vi "电机定位1.1（40M只处理采集卡）.vi"(0 "VISA I":refnum<visa-resource-name>, 1 "等待时间(ms)":u32=40, 2 "细分设置":dbl=8.0, 3 "电机急停":bool, 4 "X":dbl, 5 "精度":dbl=0.001, 6 "pulDDR2Length":u32, 8 "hDevice":i32, 10 "M-length":dbl, 12 "N-length":dbl) -> (13 "hDevice out":i32, 14 "VISA O":refnum<visa-resource-name>, 18 "X":dbl, 19 "Y":dbl)   [LabVIEW 2016]
uses:
  <vilib>/Analysis/2dsp.llb/Real FFT.vi
  <vilib>/Utility/file.llb/Write Delimited Spreadsheet (DBL).vi
  <vilib>/Utility/file.llb/Read Delimited Spreadsheet (DBL).vi
  <vilib>/Analysis/NI_AALBase.lvlib
  <vilib>/Analysis/NI_AALPro.lvlib
panel:
  out "定点积分读数":dbl
  out "有效值":dbl
  out "空扫底噪":cdb[](array[numeric])
  out "采集卡底噪":cdb[](array[numeric])
  in  "保存信号":bool
  out "幅频谱":dbl[](graph)
  out "时域谱":dbl[](graph)
  in  "查询信号":bool
  in  "Y":dbl
  in  "确定":bool
  in  "ESC":bool
  # "时域谱"
  # "频域谱"
  # "目标位置"
  # "实时位置"
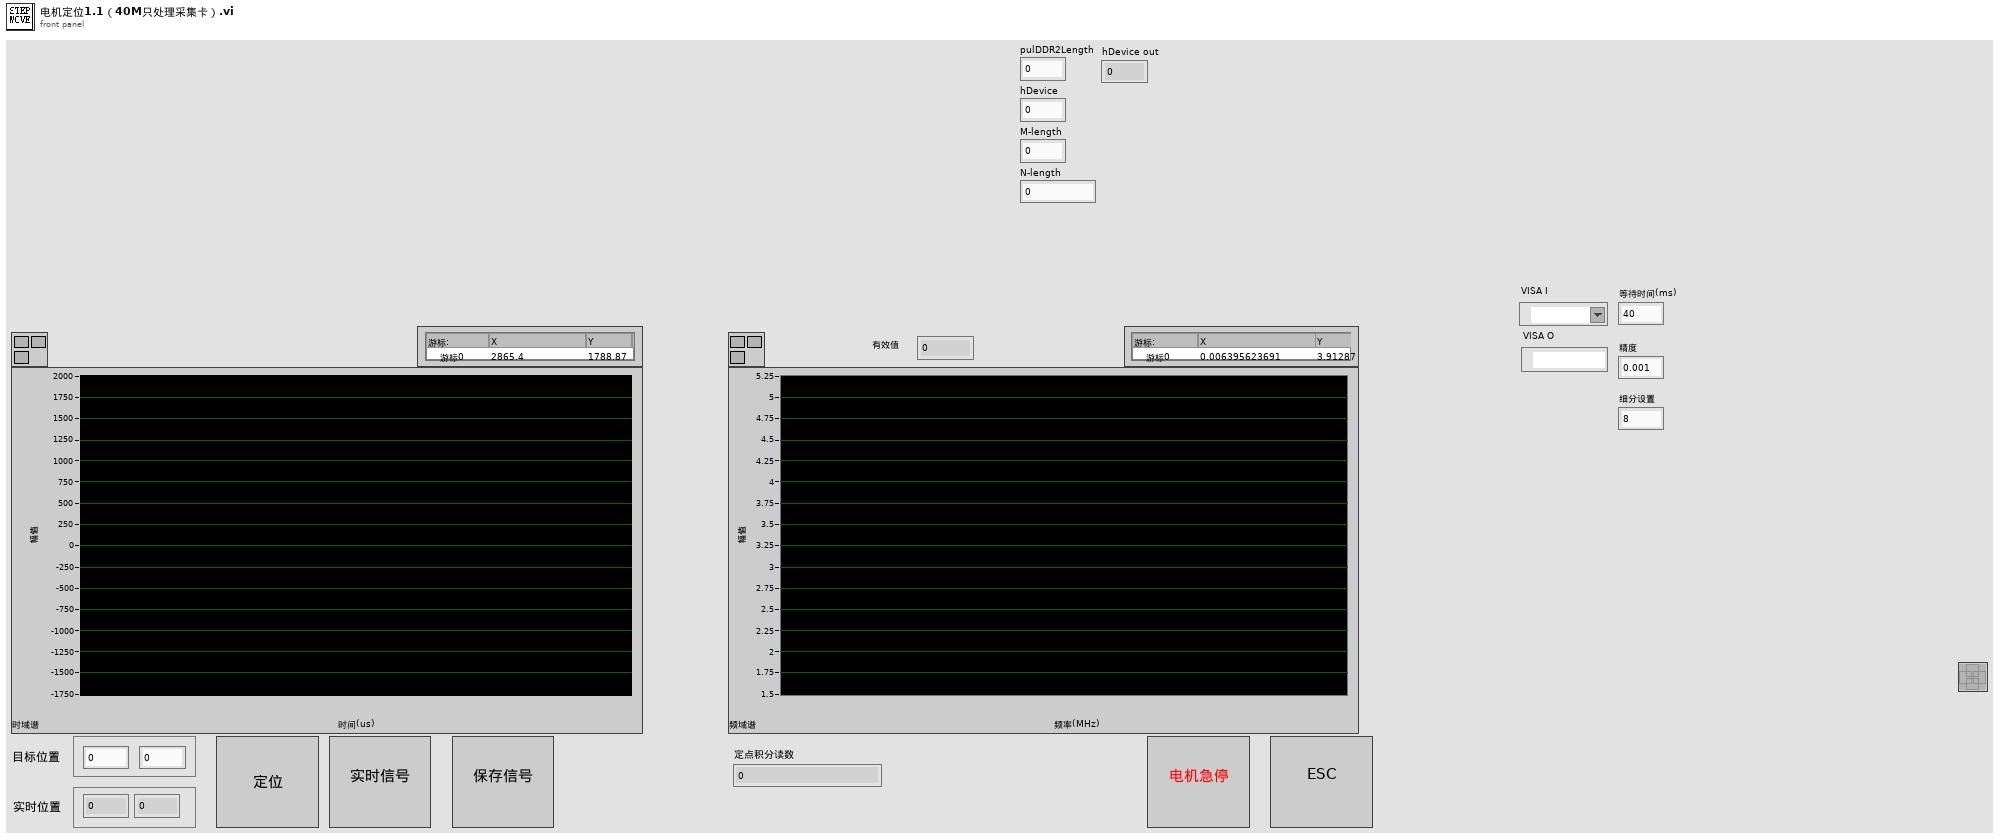
[diagram p1: front panel]
types:
  T1 = enum16{"open", "replace", "create", "open or create", "replace or create", "replace or create with confirmation"}
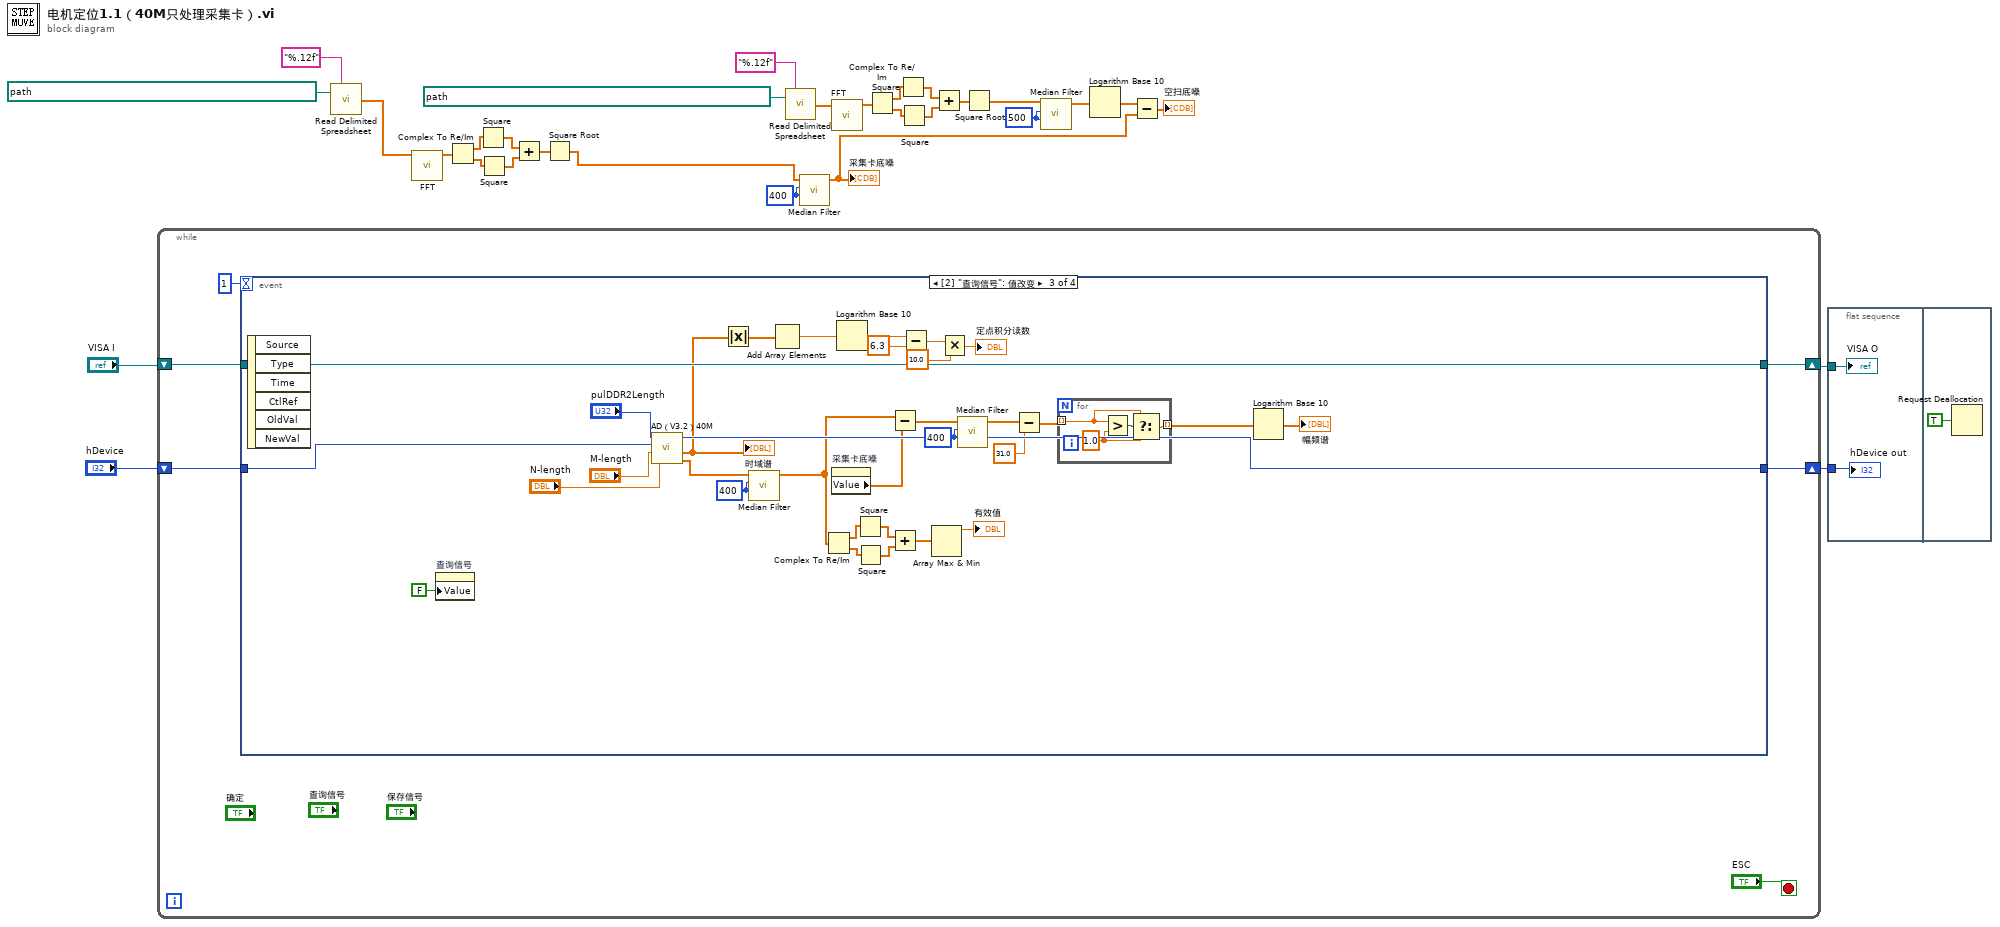
[diagram p0: block diagram]
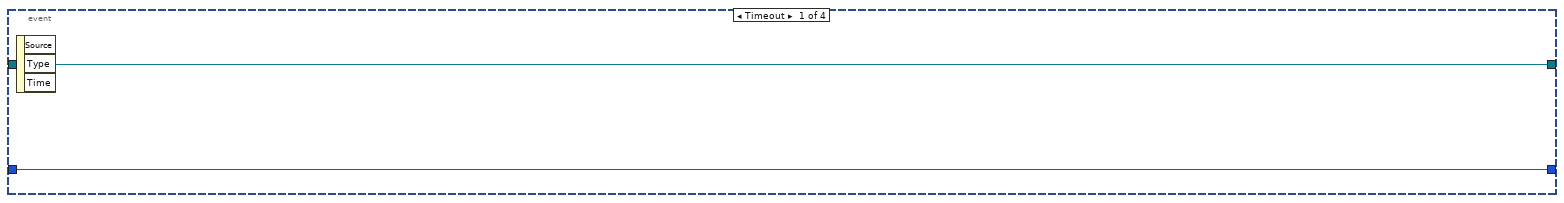
[diagram p2: hidden frame]
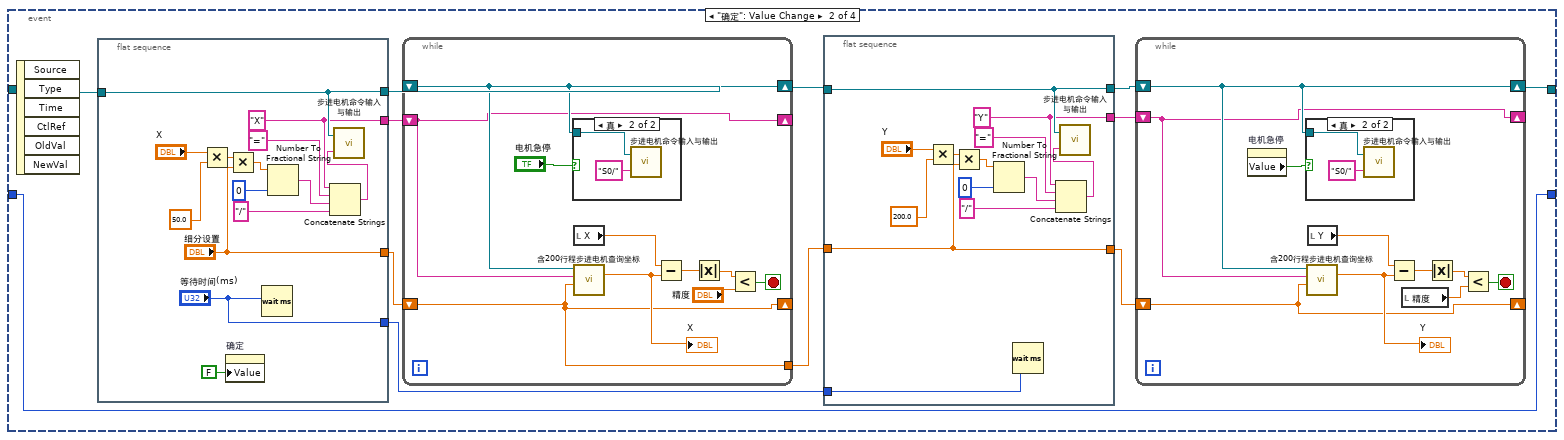
[diagram p3: hidden frame]
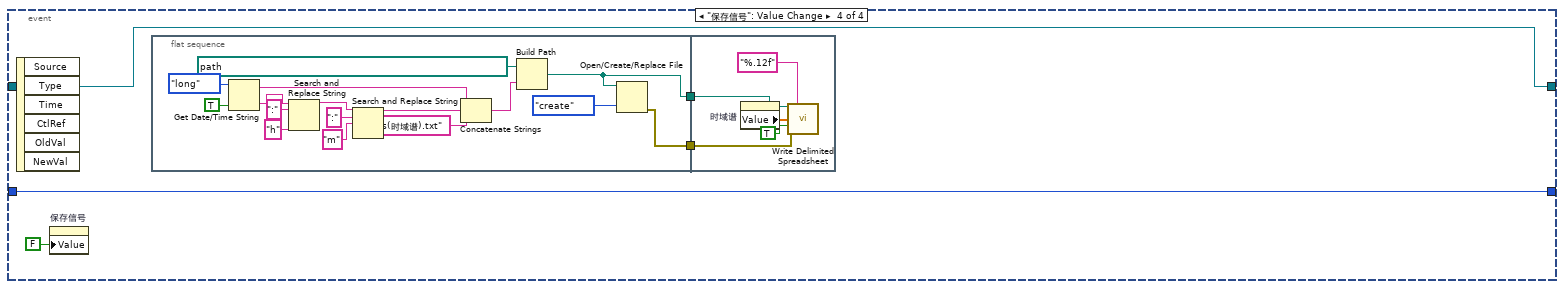
[diagram p6: hidden frame]
diagram:
  w6 = 400 ("left rank")
  w24 = 500 ("left rank")
  n1 = while {
    shift-right: [w35] -> w30
    shift-left: "VISA I" -> [w36]
    shift-right: [w32] -> w27
    shift-left: "hDevice" -> [w33]
    stop <- "ESC" stop-if-true
    n2 = event shown="[2] \"查询信号\": 值改变" {
      selector: _ -> [_ _ _ _]
      dyn-events: _ -> [_ _ _ _]
      timeout: 1 -> [_ _ _ _]
      tunnel: w36 -> [w38 w50 w133 w141]
      tunnel: [w38 w49 w133 w141] -> w35
      tunnel: w33 -> [w37 w39 w129 w140]
      tunnel: [w37 w39 w128 w140] -> w32
      event Timeout {
        n3 = event-data() -> ()  [unwired: 1 in, 3 out]
      }
      event "确定": Value Change {
        n4 = event-data() -> ()  [unwired: 1 in, 6 out]
        n5 = flat-sequence {
          tunnel: w50 -> [w93]
          tunnel: [w93] -> w48
          tunnel: ["细分设置"] -> w47
          tunnel: [w90] -> w46
          tunnel: ["等待时间(ms)"] -> w41
          frame #0 {
            w90 = "X"
            n6 = Multiply(x="X", y=50.0 ("x")) -> (x*y=w96:dbl)
            n7 = property on="确定" class="Bool (严格)"("Value"=FALSE ("确定")) -> ()  [unwired: 2 in, 2 out]
            n8 = Multiply(x=w96, y="细分设置") -> (x*y=w101:dbl)
            n9 = Wait (ms)(milliseconds to wait="等待时间(ms)") -> ()  [unwired: 1 out]
            n10 = Number To Fractional String(number=w101, precision (6)=i16 0 ("精度(6)")) -> (F-format string=w99:string)  [unwired: 2 out]
            n11 = Concatenate Strings(w90, "=" ("字符串"), w99, "/" ("字符串")) -> (w95:string)
            n12 = call "步进电机命令输入与输出.vi"("输入字符串"=w95, "串口通信端口"=w93) -> ()  [unwired: 1 out]
          }
        }
        n13 = while {
          tunnel: [w76] -> w40
          shift-right: [w82] -> w42
          shift-left: w48 -> [w82]
          shift-right: [w77] -> _
          shift-left: w46 -> [w77]
          shift-right: [w76] -> _
          shift-left: w47 -> [w76]
          stop <- w85 stop-if-true
          n14 = case shown="真" "电机急停" {
            tunnel: w82 -> [_ w86]
            frame False {
            }
            frame True {
              n15 = call "步进电机命令输入与输出.vi"("输入字符串"="S0/", "串口通信端口"=w86) -> ()  [unwired: 1 out]
            }
          }
          n16 = local read "X"() -> (w80:dbl)
          n17 = call "含200行程步进电机查询坐标.vi"("细分设置"=w76, "查询坐标轴"=w77, "串口通信端口"=w82) -> ("坐标(mm)"=w79:dbl)  [unwired: 8 in]
          "X" <- w79
          n18 = Subtract(x=w80, y=w79) -> (x-y=w84:dbl)
          n19 = Absolute Value(x=w84) -> (abs(x)=w83:dbl)
          n20 = Less?(x=w83, y="精度") -> (x < y?=w85:bool)
        }
        n21 = flat-sequence {
          tunnel: w42 -> [w67]
          tunnel: [w67] -> w45
          tunnel: [w63] -> w44
          tunnel: [w65] -> w43
          tunnel: w41 -> [w64]
          tunnel: w40 -> [w63]
          frame #0 {
            w65 = "Y"
            n22 = Multiply(x="Y", y=200.0 ("x")) -> (x*y=w70:dbl)
            n23 = Multiply(x=w70, y=w63) -> (x*y=w75:dbl)
            n24 = Number To Fractional String(number=w75, precision (6)=i16 0 ("精度(6)")) -> (F-format string=w73:string)  [unwired: 2 out]
            n25 = Wait (ms)(milliseconds to wait=w64) -> ()  [unwired: 1 out]
            n26 = Concatenate Strings(w65, "=" ("字符串"), w73, "/" ("字符串")) -> (w69:string)
            n27 = call "步进电机命令输入与输出.vi"("输入字符串"=w69, "串口通信端口"=w67) -> ()  [unwired: 1 out]
          }
        }
        n28 = while {
          shift-right: [w57] -> w49
          shift-left: w45 -> [w57]
          shift-right: [w52] -> _
          shift-left: w43 -> [w52]
          shift-right: [w51] -> _
          shift-left: w44 -> [w51]
          stop <- w60 stop-if-true
          n29 = property on="电机急停" class="Bool (严格)"() -> ("Value"=w53:bool)  [unwired: 2 in, 2 out]
          n30 = case shown="真" w53 {
            tunnel: w57 -> [_ w61]
            frame False {
            }
            frame True {
              n31 = call "步进电机命令输入与输出.vi"("输入字符串"="S0/", "串口通信端口"=w61) -> ()  [unwired: 1 out]
            }
          }
          n32 = call "含200行程步进电机查询坐标.vi"("细分设置"=w51, "查询坐标轴"=w52, "串口通信端口"=w57) -> ("坐标(mm)"=w55:dbl)  [unwired: 8 in]
          "Y" <- w55
          n33 = local read "Y"() -> (w56:dbl)
          n34 = Subtract(x=w56, y=w55) -> (x-y=w59:dbl)
          n35 = local read "精度"() -> (w54:dbl)
          n36 = Absolute Value(x=w59) -> (abs(x)=w58:dbl)
          n37 = Less?(x=w58, y=w54) -> (x < y?=w60:bool)
        }
      }
      event "查询信号": Value Change {
        w116 = 400 ("left rank")
        w126 = 400 ("left rank")
        n38 = event-data() -> ()  [unwired: 1 in, 6 out]
        n39 = property on="查询信号" class="Bool (严格)"("Value"=FALSE ("查询信号")) -> ()  [unwired: 2 in, 2 out]
        n40 = call "AD（V3.2）40M.vi"("N-length"="N-length", "M-length"="M-length", "hDevice"=w129, "pulDDR2Length"="pulDDR2Length") -> ("幅频谱"=w118:dbl[], "时域谱"=w109:dbl[], "hDevice out"=w128:i32)  [unwired: 5 in]
        "时域谱" <- w109
        n41 = Absolute Value(x=w109) -> (abs(x)=w108:dbl[])
        n42 = call <vilib>:"Median Filter.vi"("right rank"=w126, "left rank"=w126, "X"=w118) -> ("Filtered X"=w117:dbl[])  [unwired: 7 in, 1 out]
        n43 = Add Array Elements(numeric array=w108) -> (sum=w107:dbl)
        n44 = Complex To Re/Im(x + iy=w117) -> (x=w122:dbl[], y=w123:dbl[])
        n45 = property on="采集卡底噪" class="Arr (严格)"() -> ("Value"=w119:cdb[])  [unwired: 2 in, 2 out]
        n46 = Logarithm Base 10(1:w107) -> (0:w106:dbl)
        n47 = Square(x=w122) -> (x^2=w124:dbl[])
        n48 = Square(x=w123) -> (x^2=w125:dbl[])
        n49 = Subtract(x=w117, y=w119) -> (x-y=w115:cdb[])
        n50 = Add(x=w124, y=w125) -> (x+y=w121:dbl[])
        n51 = Subtract(x=w106, y=6.3) -> (x-y=w104:dbl)
        n52 = Array Max & Min(array=w121) -> (max value=→"有效值":dbl)  [unwired: 3 out]
        n53 = Multiply(x=w104, y=10.0) -> (x*y=→"定点积分读数":dbl)
        n54 = call <vilib>:"Median Filter.vi"("right rank"=w116, "left rank"=w116, "X"=w115) -> ("Filtered X"=w112:dbl[])  [unwired: 7 in, 1 out]
        n55 = Subtract(x=w112, y=31.0) -> (x-y=w113:dbl[])
        n56 = for {
          tunnel: w113 -> [w135] mode=indexing
          tunnel: [w136] -> w114 mode=indexing
          w134 = 1.0
          n57 = Greater?(x=w135, y=w134) -> (0:w137:bool)
          n58 = Select(t=w135, s=w137, f=w134) -> (s? t:f=w136:dbl)
        }
        n59 = Logarithm Base 10(1:w114) -> (0:→"幅频谱":dbl[])
      }
      event "保存信号": Value Change {
        n60 = event-data() -> ()  [unwired: 1 in, 6 out]
        n61 = property on="保存信号" class="Bool (严格)"("Value"=FALSE ("保存信号")) -> ()  [unwired: 2 in, 2 out]
        n62 = flat-sequence {
          tunnel: [w156] -> w139
          tunnel: [w155] -> w138
          tunnel: w139 -> [w160]
          tunnel: w138 -> [w159]
          frame #0 {
            n63 = Get Date/Time String(date format (0)=enum16{"short", "long", "abbreviated"}."long" ("日期格式(0)"), want seconds? (F)=TRUE ("需要秒？(F)")) -> (date string=w147:string, time string=w148:string)  [unwired: 1 in]
            n64 = Search and Replace String(input string=w148, search string=":" ("搜索字符串"), replace string="h" ("替换字符串(\"\")")) -> (result string=w153:string)  [unwired: 5 in, 3 out]
            n65 = Search and Replace String(input string=w153, search string=":" ("搜索字符串"), replace string="m" ("替换字符串(\"\")")) -> (result string=w146:string)  [unwired: 5 in, 3 out]
            n66 = Concatenate Strings(w147, w146, "s(时域谱).txt" ("字符串")) -> (w145:string)
            n67 = Build Path(base path=path "C:/Users/H301/Desktop/art采集实验数据/单点时域谱" ("基路径"), name or relative path=w145) -> (appended path=w156:path)
            n68 = Open/Create/Replace File(file path (use dialog)=w156, operation (0:open)=T1."create" ("操作(0:open)")) -> (error out=w155:errorcluster)  [unwired: 4 in, 2 out]
          }
          frame #1 {
            n69 = property on="时域谱" class="WFGraph (严格)"() -> ("Value"=w161:dbl[])  [unwired: 2 in, 2 out]
            n70 = call-poly <vilib>:"Write Delimited Spreadsheet.vi"("file path (dialog if empty)"=w160, "format (%.3f)"="%.12f", "1D data"=w161, "append to file? (new file:F)"=TRUE, "error in (no error)"=w159) -> ()  [unwired: 9 in, 2 out]
          }
        }
      }
    }
  }
  n71 = call-poly <vilib>:"Read Delimited Spreadsheet.vi"("file path (dialog if empty)"=path "C:/Users/H301/Desktop/art采集实验数据/2018年7月17日9h55m04s(采集卡底噪).txt", "format (%.3f)"="%.12f") -> ("first row"=w7:dbl[])  [unwired: 8 in, 5 out]
  n72 = call-poly <vilib>:"FFT.vi"("X"=w7) -> ("FFT {X}"=w10:cdb[])  [unwired: 9 in, 1 out]
  n73 = Complex To Re/Im(x + iy=w10) -> (x=w8:dbl[], y=w9:dbl[])
  n74 = Square(x=w8) -> (x^2=w11:dbl[])
  n75 = Square(x=w9) -> (x^2=w12:dbl[])
  n76 = Add(x=w11, y=w12) -> (x+y=w13:dbl[])
  n77 = Square Root(x=w13) -> (sqrt(x)=w1:dbl[])
  n78 = call-poly <vilib>:"Read Delimited Spreadsheet.vi"("file path (dialog if empty)"=path "C:/Users/H301/Desktop/art采集实验数据/信号源均值底噪.txt", "format (%.3f)"="%.12f") -> ("first row"=w23:dbl[])  [unwired: 8 in, 5 out]
  n79 = call <vilib>:"Median Filter.vi"("right rank"=w6, "left rank"=w6, "X"=w1) -> ("Filtered X"=w3:dbl[])  [unwired: 7 in, 1 out]
  "采集卡底噪" <- w3
  n80 = call-poly <vilib>:"FFT.vi"("X"=w23) -> ("FFT {X}"=w18:cdb[])  [unwired: 9 in, 1 out]
  n81 = Complex To Re/Im(x + iy=w18) -> (x=w20:dbl[], y=w19:dbl[])
  n82 = Square(x=w20) -> (x^2=w17:dbl[])
  n83 = Square(x=w19) -> (x^2=w16:dbl[])
  n84 = Add(x=w17, y=w16) -> (x+y=w15:dbl[])
  n85 = Square Root(x=w15) -> (sqrt(x)=w14:dbl[])
  n86 = call <vilib>:"Median Filter.vi"("right rank"=w24, "left rank"=w24, "X"=w14) -> ("Filtered X"=w5:dbl[])  [unwired: 7 in, 1 out]
  n87 = Logarithm Base 10(1:w5) -> (0:w4:dbl[])
  n88 = Subtract(x=w4, y=w3) -> (x-y=→"空扫底噪":dbl[])
  n89 = flat-sequence {
    tunnel: w30 -> [w165]
    tunnel: w27 -> [w164]
    frame #0 {
      "VISA O" <- w165
      "hDevice out" <- w164
    }
    frame #1 {
      n90 = Request Deallocation(TRUE ("标志")) -> ()
    }
  }
